vi "CRYPreview InsDel.vi"(10 "Graph VI Ref":refnum<vi>, 11 "sAction":string) -> ()   [LabVIEW 2013]
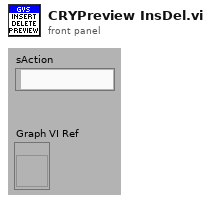
[diagram p1: front panel]
types:
  T1 = typedef "LVBoundsTypeDef.ctl" = cluster{"Width":u32, "Height":u32}
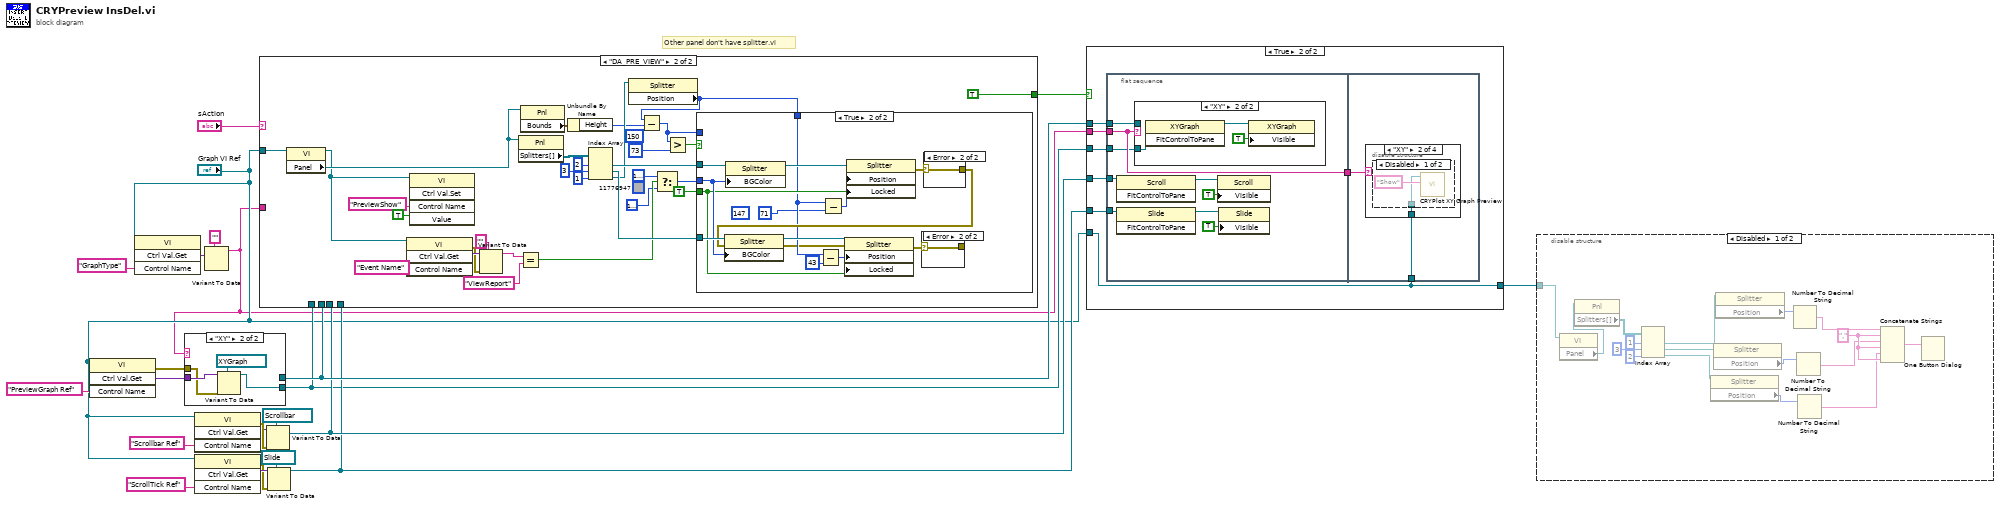
[diagram p0: block diagram]
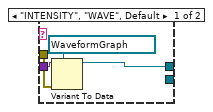
[diagram p3: hidden frame]
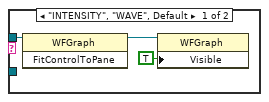
[diagram p5: hidden frame]
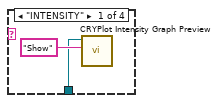
[diagram p6: hidden frame]
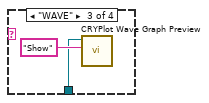
[diagram p8: hidden frame]
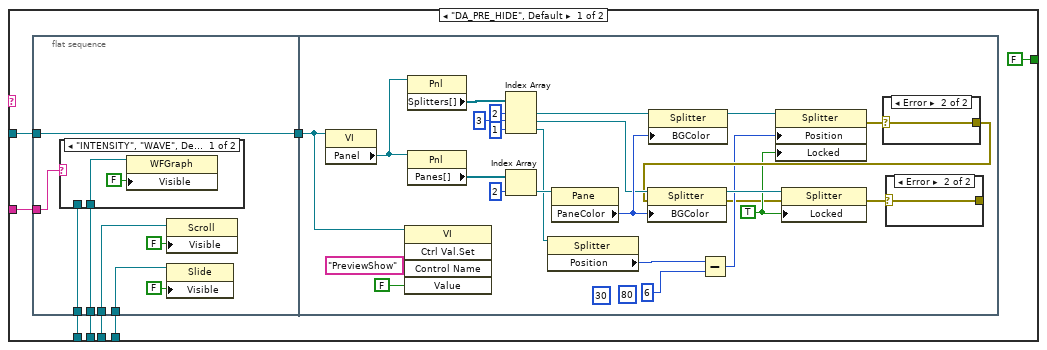
[diagram p10: hidden frame]
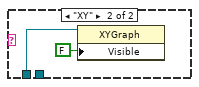
[diagram p11: hidden frame]
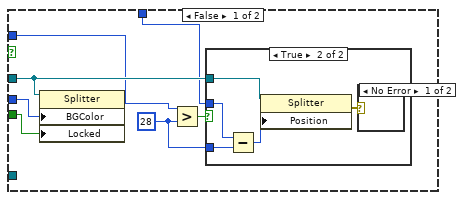
[diagram p14: hidden frame]
diagram:
  # "Other panel don't have splitter.vi"
  n1 = invoke class="VI" method="Ctrl Val.Get"(reference="Graph VI Ref", "Control Name"="PreviewGraph Ref") -> (error out=w21:errorcluster, "Get Control Value Variant"=w22:variant)  [unwired: 2 in, 2 out]
  n2 = invoke class="VI" method="Ctrl Val.Get"(reference="Graph VI Ref", "Control Name"="GraphType") -> ("Get Control Value Variant"=w3:variant)  [unwired: 2 in, 3 out]
  n3 = invoke class="VI" method="Ctrl Val.Get"(reference="Graph VI Ref", "Control Name"="Scrollbar Ref") -> (error out=w17:errorcluster, "Get Control Value Variant"=w16:variant)  [unwired: 2 in, 2 out]
  n4 = invoke class="VI" method="Ctrl Val.Get"(reference="Graph VI Ref", "Control Name"="ScrollTick Ref") -> (error out=w14:errorcluster, "Get Control Value Variant"=w15:variant)  [unwired: 2 in, 2 out]
  n5 = Variant To Data(type="" ("Control Name"), Variant=w3) -> (data=w1:string)  [unwired: 1 in, 1 out]
  n6 = case shown="\"XY\"" w1 {
    tunnel: w22 -> [w27 w31]
    tunnel: w21 -> [w26 w30]
    tunnel: [w24 _] -> w10
    tunnel: [_ w28] -> w7
    frame "INTENSITY", "WAVE", Default {
      n7 = Variant To Data(error in=w26, type=refnum<vi> refnum ("Legend Ref"), Variant=w27) -> (data=w24:refnum<vi>)  [unwired: 1 out]
    }
    frame "XY" {
      n8 = Variant To Data(error in=w30, type=refnum<vi> refnum ("Legend Ref"), Variant=w31) -> (data=w28:refnum<vi>)  [unwired: 1 out]
    }
  }
  n9 = Variant To Data(error in=w17, type=refnum<vi> refnum ("Legend Ref"), Variant=w16) -> (data=w9:refnum<vi>)  [unwired: 1 out]
  n10 = Variant To Data(error in=w14, type=refnum<vi> refnum ("Legend Ref"), Variant=w15) -> (data=w8:refnum<vi>)  [unwired: 1 out]
  n11 = case shown="\"DA_PRE_VIEW\"" "sAction" {
    tunnel: "Graph VI Ref" -> [w38 w106]
    tunnel: [FALSE TRUE] -> w11
    tunnel: w10 -> [w36 _]
    tunnel: w9 -> [w35 _]
    tunnel: w8 -> [w34 _]
    tunnel: w7 -> [w33 _]
    tunnel: w1 -> [w32 _]
    frame "DA_PRE_HIDE", Default {
      n12 = flat-sequence {
        tunnel: w38 -> [w47]
        tunnel: [w47] -> w37
        tunnel: w36 -> [w44]
        tunnel: w35 -> [w43]
        tunnel: w34 -> [w42]
        tunnel: w33 -> [w40]
        tunnel: w32 -> [w41]
        tunnel: w37 -> [w52]
        frame #0 {
          n13 = case shown="\"INTENSITY\", \"WAVE\", Default" w41 {
            tunnel: w44 -> [w48 _]
            tunnel: w40 -> [_ w50]
            frame "INTENSITY", "WAVE", Default {
              n14 = property class="WFGraph"(reference=w48, "Visible"=FALSE) -> ()  [unwired: 1 in, 2 out]
            }
            frame "XY" {
              n15 = property class="XYGraph"(reference=w50, "Visible"=FALSE) -> ()  [unwired: 1 in, 2 out]
            }
          }
          n16 = property class="Scroll"(reference=w43, "Visible"=FALSE) -> ()  [unwired: 1 in, 2 out]
          n17 = property class="Slide"(reference=w42, "Visible"=FALSE) -> ()  [unwired: 1 in, 2 out]
        }
        frame #1 {
          (unwired) u32 30 ("y")
          w57 = TRUE ("Splitter Position Locked")
          (unwired) u32 80 ("y")
          n18 = property class="VI"(reference=w52) -> ("Panel"=w75:refnum<vi>)  [unwired: 1 in, 2 out]
          n19 = invoke class="VI" method="Ctrl Val.Set"(reference=w52, "Control Name"="PreviewShow", "Value"=FALSE ("Visible")) -> ()  [unwired: 2 in, 5 out]
          n20 = property class="Pnl"(reference=w75) -> ("Splitters[]"=w71:refnum<vi>[])  [unwired: 1 in, 2 out]
          n21 = property class="Pnl"(reference=w75) -> ("Panes[]"=w69:refnum<vi>[])  [unwired: 1 in, 2 out]
          n22 = Index Array(array=w71, index #1=2 ("index"), index #2=3 ("index"), index #3=1 ("index")) -> (element #1=w64:refnum<vi>, element #2=w63:refnum<vi>, element #3=w65:refnum<vi>)
          n23 = Index Array(array=w69, index=2) -> (element=w72:refnum<vi>)
          n24 = property on="Property Node" class="Splitter"(reference=w65) -> ("Position"=w59:i32)  [unwired: 1 in, 2 out]
          n25 = property class="Pane"(reference=w72) -> ("PaneColor"=w67:u32)  [unwired: 1 in, 2 out]
          n26 = property on="Property Node" class="Splitter"(reference=w64, "BGColor"=w67) -> (reference out=w73:refnum<vi>)  [unwired: 1 in, 1 out]
          n27 = Subtract(x=w59, y=u32 6) -> (x-y=w58:u32)
          n28 = property on="Property Node" class="Splitter"(reference=w73, "Position"=w58, "Locked"=w57) -> (error out=w74:errorcluster)  [unwired: 1 in, 1 out]
          n29 = case shown="Error" w74 {
            selector: w74 -> [w79 w80]
            tunnel: [w79 w80] -> w60
            frame No Error {
            }
            frame Error {
            }
          }
          n30 = property on="Property Node" class="Splitter"(reference=w63, error in=w60, "BGColor"=w67) -> (reference out=w62:refnum<vi>, error out=w56:errorcluster)
          n31 = property on="Property Node" class="Splitter"(reference=w62, error in=w56, "Locked"=w57) -> (error out=w61:errorcluster)  [unwired: 1 out]
          n32 = case shown="Error" w61 {
            selector: w61 -> [w77 w78]
            tunnel: [w77 w78] -> _
            frame No Error {
            }
            frame Error {
            }
          }
        }
      }
    }
    frame "DA_PRE_VIEW" {
      (unwired) u32 11776947
      (unwired) u32 150 ("y")
      n33 = property class="VI"(reference=w106) -> (reference out=w85:refnum<vi>, "Panel"=w108:refnum<vi>)  [unwired: 1 in, 1 out]
      n34 = invoke class="VI" method="Ctrl Val.Get"(reference=w85, "Control Name"="Event Name") -> (error out=w88:errorcluster, "Get Control Value Variant"=w89:variant)  [unwired: 2 in, 2 out]
      n35 = invoke class="VI" method="Ctrl Val.Set"(reference=w85, "Control Name"="PreviewShow", "Value"=TRUE ("Visible")) -> ()  [unwired: 2 in, 5 out]
      n36 = Variant To Data(error in=w88, type="" ("Control Name"), Variant=w89) -> (data=w90:string)  [unwired: 1 out]
      n37 = property class="Pnl"(reference=w108) -> ("Splitters[]"=w110:refnum<vi>[])  [unwired: 1 in, 2 out]
      n38 = Equal?(x=w90, y="ViewReport" ("Control Name")) -> (x = y?=w82:bool)
      n39 = property class="Pnl"(reference=w108) -> ("Bounds"=w107:T1)  [unwired: 1 in, 2 out]
      n40 = Unbundle By Name(w107) -> ("Height"=w98:u32)
      n41 = Index Array(array=w110, index #1=2 ("index"), index #2=3 ("index"), index #3=1 ("index")) -> (element #1=w105:refnum<vi>, element #2=w101:refnum<vi>, element #3=w99:refnum<vi>)
      n42 = property on="Property Node" class="Splitter"(reference=w99) -> ("Position"=w97:i32)  [unwired: 1 in, 2 out]
      n43 = Subtract(x=w97, y=w98) -> (x-y=w96:u32)
      n44 = Select(t=u32 16777226, s=w82, f=u32 16777238) -> (s? t:f=w83:u32)
      n45 = Greater?(x=w96, y=u32 73) -> (0:w95:bool)
      n46 = case shown="True" w95 {
        tunnel: w105 -> [w114 w137]
        tunnel: w83 -> [w117 w134]
        tunnel: TRUE ("Splitter Position Locked") -> [w116 w133]
        tunnel: w101 -> [_ w135]
        tunnel: w97 -> [w111 w125]
        tunnel: w96 -> [w112 _]
        frame False {
          w113 = u32 28 ("y")
          n47 = property on="Property Node" class="Splitter"(reference=w114, "BGColor"=w117, "Locked"=w116) -> ()  [unwired: 1 in, 2 out]
          n48 = Greater?(x=w112, y=w113) -> (0:w115:bool)
          n49 = case shown="True" w115 {
            tunnel: w114 -> [_ w122]
            tunnel: w111 -> [_ w121]
            tunnel: w113 -> [_ w119]
            frame False {
            }
            frame True {
              n50 = Subtract(x=w121, y=w119) -> (x-y=w120:u32)
              n51 = property on="Property Node" class="Splitter"(reference=w122, "Position"=w120) -> (error out=w118:errorcluster)  [unwired: 1 in, 1 out]
              n52 = case shown="No Error" w118 {
                frame No Error {
                }
                frame Error {
                }
              }
            }
          }
        }
        frame True {
          (unwired) u32 147 ("y")
          n53 = property on="Property Node" class="Splitter"(reference=w137, "BGColor"=w134) -> (reference out=w131:refnum<vi>)  [unwired: 1 in, 1 out]
          n54 = Subtract(x=w125, y=u32 43) -> (x-y=w128:u32)
          n55 = Subtract(x=w125, y=u32 71) -> (x-y=w136:u32)
          n56 = property on="Property Node" class="Splitter"(reference=w131, "Position"=w136, "Locked"=w133) -> (error out=w132:errorcluster)  [unwired: 1 in, 1 out]
          n57 = case shown="Error" w132 {
            selector: w132 -> [w140 w141]
            tunnel: [w140 w141] -> w126
            frame No Error {
            }
            frame Error {
            }
          }
          n58 = property on="Property Node" class="Splitter"(reference=w135, error in=w126, "BGColor"=w134) -> (reference out=w127:refnum<vi>, error out=w123:errorcluster)
          n59 = property on="Property Node" class="Splitter"(reference=w127, error in=w123, "Position"=w128, "Locked"=w133) -> (error out=w130:errorcluster)  [unwired: 1 out]
          n60 = case shown="Error" w130 {
            selector: w130 -> [w138 w139]
            tunnel: [w138 w139] -> _
            frame No Error {
            }
            frame Error {
            }
          }
        }
      }
    }
  }
  n61 = case shown="True" w11 {
    tunnel: w10 -> [_ w149]
    tunnel: w9 -> [_ w148]
    tunnel: w8 -> [_ w147]
    tunnel: "Graph VI Ref" -> [w142 w143]
    tunnel: w1 -> [_ w146]
    tunnel: w7 -> [_ w144]
    tunnel: [w142 w143] -> w6
    frame False {
    }
    frame True {
      n62 = flat-sequence {
        tunnel: w149 -> [w158]
        tunnel: w148 -> [w153]
        tunnel: w147 -> [w152]
        tunnel: w146 -> [w151]
        tunnel: [w151] -> w145
        tunnel: w144 -> [w150]
        tunnel: w143 -> [w166]
        tunnel: w145 -> [w165]
        frame #0 {
          n63 = invoke class="Scroll" method="FitControlToPane"(reference=w153) -> (reference out=w157:refnum<vi>)  [unwired: 2 in, 2 out]
          n64 = invoke class="Slide" method="FitControlToPane"(reference=w152) -> (reference out=w154:refnum<vi>)  [unwired: 2 in, 2 out]
          n65 = case shown="\"XY\"" w151 {
            tunnel: w158 -> [w161 _]
            tunnel: w150 -> [_ w162]
            frame "INTENSITY", "WAVE", Default {
              n66 = invoke class="WFGraph" method="FitControlToPane"(reference=w161) -> (reference out=w159:refnum<vi>)  [unwired: 2 in, 2 out]
              n67 = property class="WFGraph"(reference=w159, "Visible"=TRUE) -> ()  [unwired: 1 in, 2 out]
            }
            frame "XY" {
              n68 = invoke class="XYGraph" method="FitControlToPane"(reference=w162) -> (reference out=w163:refnum<vi>)  [unwired: 2 in, 2 out]
              n69 = property class="XYGraph"(reference=w163, "Visible"=TRUE) -> ()  [unwired: 1 in, 2 out]
            }
          }
          n70 = property class="Scroll"(reference=w157, "Visible"=TRUE) -> ()  [unwired: 1 in, 2 out]
          n71 = property class="Slide"(reference=w154, "Visible"=TRUE) -> ()  [unwired: 1 in, 2 out]
        }
        frame #1 {
          n72 = case shown="\"XY\"" w165 {
            tunnel: w166 -> [w167 w169 w172 _]
            frame "INTENSITY" {
              n73 = call "CRYPlot Intensity Graph Preview.vi"("sOption"="Show", "IntensityGraph VI Ref"=w167) -> ()  [unwired: 10 in]
            }
            frame "XY" {
              n74 = disable-structure shown="Disabled" {
                disable-tunnel: w169 -> [w170 _]
                frame Disabled {
                  n75 = call "CRYPlot XY Graph Preview.vi"("sOption"="Show", "Graph VI Ref"=w170) -> ()  [unwired: 10 in]
                }
                frame Enabled {
                }
              }
            }
            frame "WAVE" {
              n76 = call "CRYPlot Wave Graph Preview.vi"("sOption"="Show", "Graph VI Ref"=w172) -> ()  [unwired: 10 in]
            }
            frame Default {
            }
          }
        }
      }
    }
  }
  n77 = disable-structure shown="Disabled" {
    disable-tunnel: w6 -> [w187 _]
    frame Disabled {
      w177 = "," ("string")
      n78 = property class="VI"(reference=w187) -> ("Panel"=w186:refnum<vi>)  [unwired: 1 in, 2 out]
      n79 = property class="Pnl"(reference=w186) -> ("Splitters[]"=w185:refnum<vi>[])  [unwired: 1 in, 2 out]
      n80 = Index Array(array=w185, index #1=1 ("index"), index #2=3 ("index"), index #3=2 ("index")) -> (element #1=w184:refnum<vi>, element #2=w183:refnum<vi>, element #3=w182:refnum<vi>)
      n81 = property on="Property Node" class="Splitter"(reference=w182) -> ("Position"=w179:i32)  [unwired: 1 in, 2 out]
      n82 = property on="Property Node" class="Splitter"(reference=w183) -> ("Position"=w180:i32)  [unwired: 1 in, 2 out]
      n83 = property on="Property Node" class="Splitter"(reference=w184) -> ("Position"=w181:i32)  [unwired: 1 in, 2 out]
      n84 = Number To Decimal String(number=w181) -> (decimal integer string=w178:string)  [unwired: 1 in]
      n85 = Number To Decimal String(number=w180) -> (decimal integer string=w176:string)  [unwired: 1 in]
      n86 = Number To Decimal String(number=w179) -> (decimal integer string=w175:string)  [unwired: 1 in]
      n87 = Concatenate Strings(w178, w177, w176, w177, w175, w177) -> (w174:string)
      n88 = One Button Dialog(message=w174) -> ()  [unwired: 1 in, 1 out]
    }
    frame Enabled {
    }
  }
